vi "Write XBox Controller Config.vi"(8 "error in (no error)":errorcluster, 10 "XBox One Controller Config":T1, 11 "Comp XBox One Controller in":refnum<class "Comp XBox One Controller.lvclass">) -> (0 "error out":errorcluster, 3 "Comp XBox One Controller out":refnum<class "Comp XBox One Controller.lvclass">)   [LabVIEW 2014, in "Comp XBox One Controller.lvlib" / "Comp XBox One Controller.lvclass"]
uses:
  Comp XBox One Controller.lvclass
  Comp X1 Config.ctl
  <vilib>/Rock Robotics/WPI/Joystick/WPI_JoystickDeviceEnum.ctl
  Comp XBox One Controller.lvclass/Comp XBox One Controller.ctl
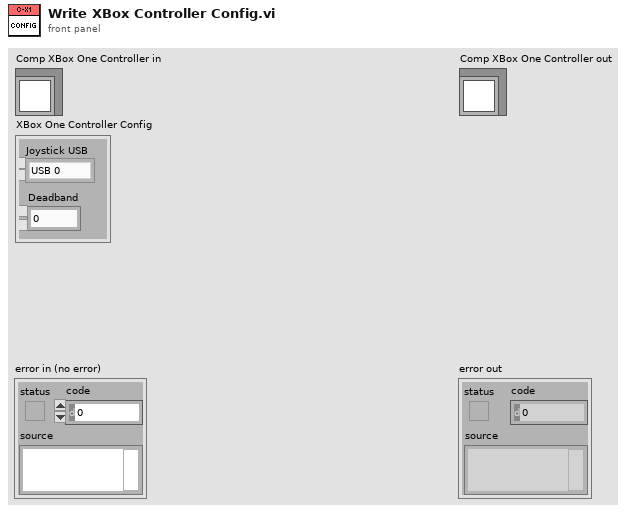
[diagram p1: front panel]
types:
  T1 = typedef "Comp XBox One Controller.lvlib/Comp XBox One Controller.lvclass/Comp X1 Config.ctl" = cluster{"Joystick USB":T2, "Deadband":dbl}
  T2 = typedef "WPI_JoystickDeviceEnum.ctl" = enum16{"USB 0", "USB 1", "USB 2", "USB 3", "USB 4", "USB 5"}
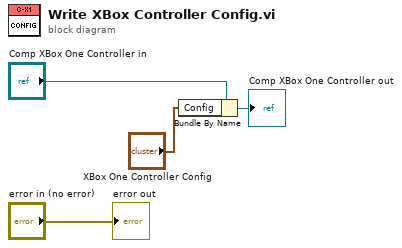
[diagram p0: block diagram]
diagram:
  n1 = Bundle By Name(cluster="Comp XBox One Controller in", "Config"="XBox One Controller Config") -> (→"Comp XBox One Controller out":refnum<class "Comp XBox One Controller.lvclass">)
  "error out" <- "error in (no error)"
